vi "AttackerPrePenalty.vi"(6 "balls":T2[](array[typedef]), 8 "Opponent goalie":T1, 9 "Field Size in":T3, 10 "Numeric":i32, 11 "Robot in":T1) -> (3 "Robot out":T1)   [LabVIEW 2016]
uses:
  Core/AI Robot.ctl
  Core/Field Size.ctl
  Core/AI Ball.ctl
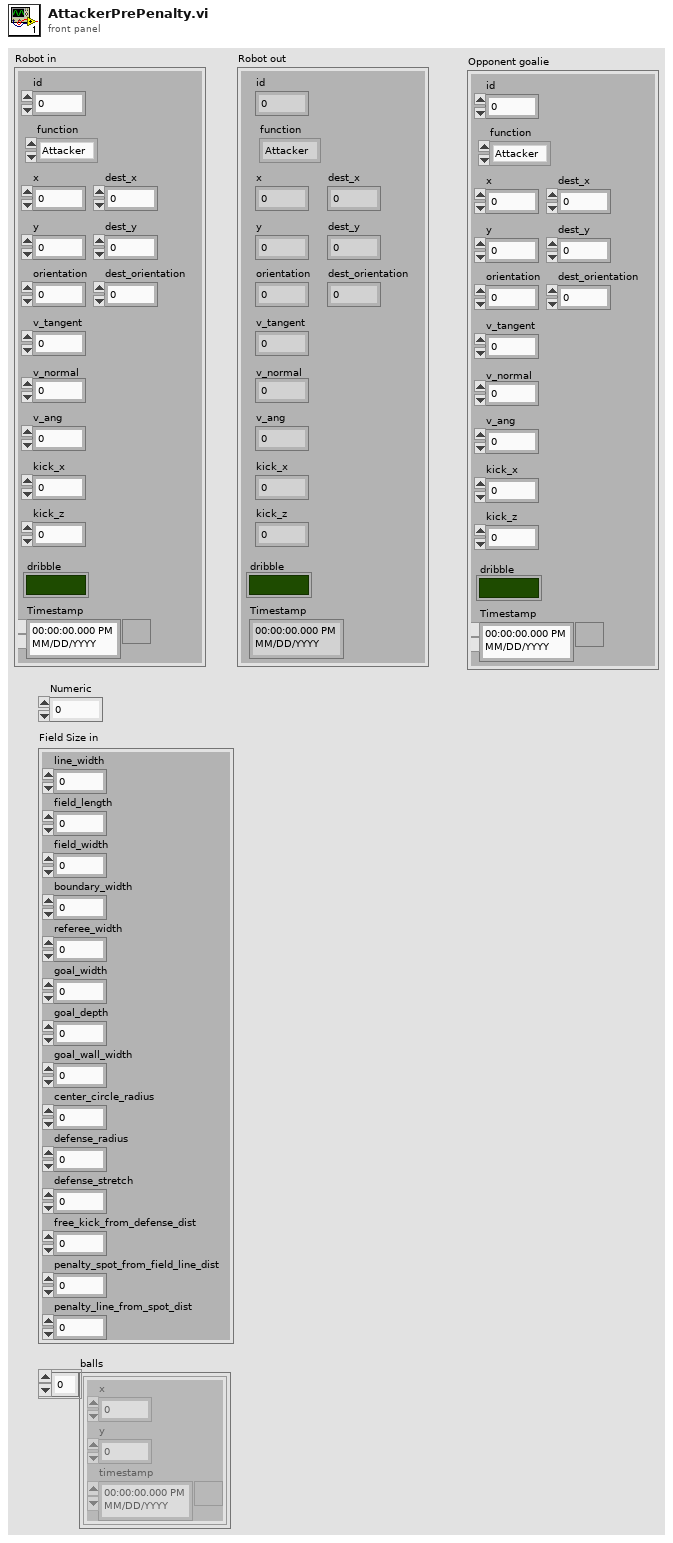
[diagram p1: front panel]
types:
  T1 = typedef "AI Robot.ctl" = cluster{"id":u32, "function":enum16{"Attacker", "Goalie", "Defender"}, "x":dbl, "y":dbl, "orientation":dbl, "v_tangent":dbl, "v_normal":dbl, "v_ang":dbl, "kick_x":dbl, "kick_z":dbl, "dribble":bool, "Timestamp":timestamp, "dest_x":dbl, "dest_y":dbl, "dest_orientation":dbl}
  T2 = typedef "AI Ball.ctl" = cluster{"x":dbl, "y":dbl, "timestamp":timestamp}
  T3 = typedef "Field Size.ctl" = cluster{"line_width":u32, "field_length":u32, "field_width":u32, "boundary_width":u32, "referee_width":u32, "goal_width":u32, "goal_depth":u32, "goal_wall_width":u32, "center_circle_radius":u32, "defense_radius":u32, "defense_stretch":u32, "free_kick_from_defense_dist":u32, "penalty_spot_from_field_line_dist":u32, "penalty_line_from_spot_dist":u32}
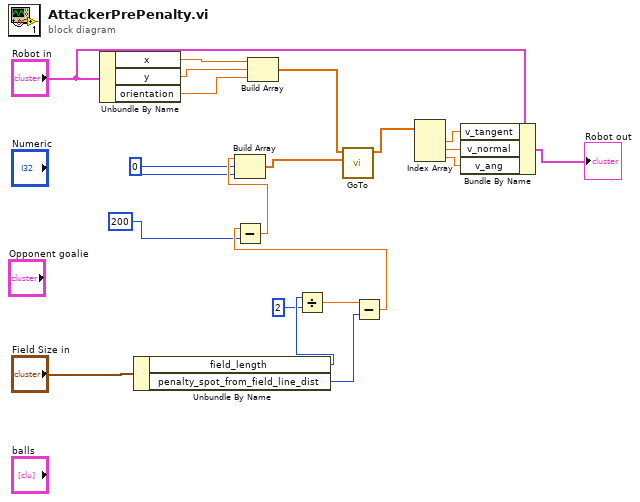
[diagram p0: block diagram]
diagram:
  w1 = u32 0 ("element")
  n1 = Unbundle By Name("Robot in") -> ("x"=w20:dbl, "y"=w19:dbl, "orientation"=w18:dbl)
  n2 = Unbundle By Name("Field Size in") -> ("field_length"=w4:u32, "penalty_spot_from_field_line_dist"=w15:u32)
  n3 = Build Array(w20, w19, w18) -> (w17:dbl[])
  n4 = Divide(x=w4, y=u32 2) -> (x/y=w2:dbl)
  n5 = Subtract(x=w2, y=w15) -> (x-y=w14:dbl)
  n6 = Subtract(x=w14, y=200) -> (x-y=w12:dbl)
  n7 = Build Array(w12, w1, w1) -> (w11:dbl[])
  n8 = call "GoTo.vi"("Target"=w11, "Position"=w17) -> ("Output\nVelocity"=w10:dbl[])  [unwired: 9 in]
  n9 = Index Array(array=w10) -> (element #1=w8:dbl, element #2=w7:dbl, element #3=w6:dbl)  [unwired: 3 in]
  n10 = Bundle By Name(cluster="Robot in", "v_tangent"=w8, "v_normal"=w7, "v_ang"=w6) -> (→"Robot out":T1)
